vi "getGain.vi"(6 "Delay between send and receive [ms]":i32=100, 8 "error in (no error)":errorcluster, 11 "CCD in":refnum<class "CCD.lvclass">) -> (0 "error out":errorcluster, 1 "token":i32, 2 "info":string, 3 "CCD out":refnum<class "CCD.lvclass">)   [LabVIEW 2023, in "CCD.lvclass"]
doc: "Gets the current gain token and the associated description information for the gain token. Gain tokens and their descriptions are part of the CCD configuration information. See ccd_getConfig command.\nFor example:\n\n\"gains\": [\n {\n \"info\": \"Best Dynamic Range\",\n \"token\": 1\n },\n {\n \"info\": \"High Sensitivity\",\n \"token\": 2\n },\n {\n \"info\": \"High Light\",\n \"token\": 0\n }\n]"
uses:
  CCD.lvclass
  CCD.lvclass/CCD.ctl
  20f7d3bd-08ac-4524-9bed-df36c1da25a0.vi
  a21955fc-e3a0-4e36-8495-41f1bfac7860.vi
  GenericDevice/GenericDevice.lvclass
  Gain.ctl
panel:
  # "Connector Pane"
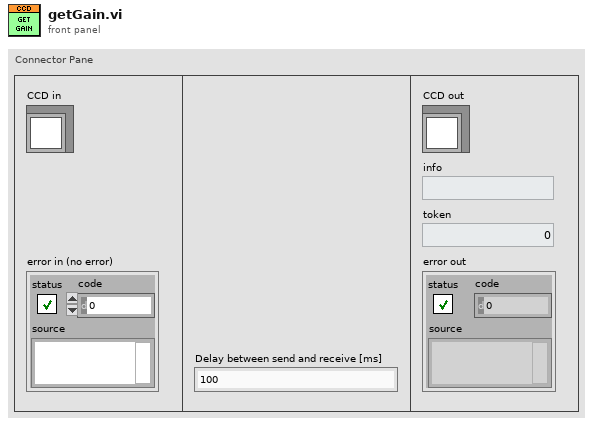
[diagram p1: front panel]
types:
  T1 = typedef "CCD.lvclass/Gain.ctl" = cluster{"info":string, "token":i32}
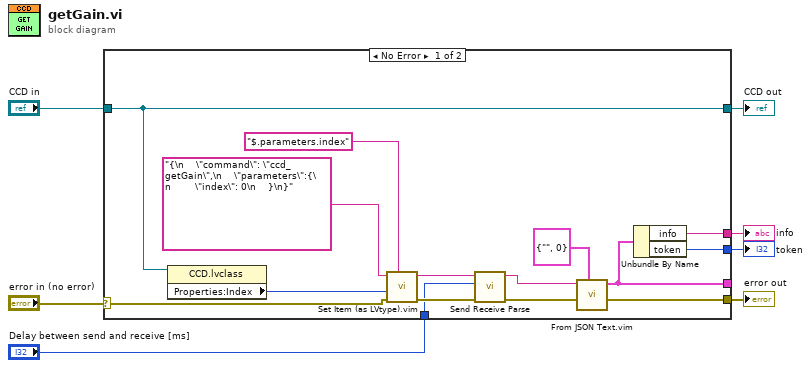
[diagram p0: block diagram]
diagram:
  n1 = case shown="No Error" "error in (no error)" {
    selector: "error in (no error)" -> [w18 w24]
    tunnel: [w17 w24] -> w6
    tunnel: [w20 w23] -> w4
    tunnel: "CCD in" -> [w20 w23]
    tunnel: [w13 _] -> _
    tunnel: [w12 _] -> w3
    tunnel: [w10 _] -> w1
    tunnel: "Delay between send and receive [ms]" -> [w11 _]
    frame No Error {
      n2 = property class="CCD.lvclass"(reference=w20) -> ("Properties:Index"=w19:i32)  [unwired: 1 in, 2 out]
      n3 = call "Set Item (as LVtype).vim"("$Path or Item Name"="$.parameters.index", "error in (no error)"=w18, "Anything"=w19, "JSON"="{\n    \"command\": \"ccd_getGain\",\n    \"parameters\":{\n        \"index\": 0\n    }\n}") -> ("error out"=w14:errorcluster, "<JSON>"=w8:string)  [unwired: 4 in, 1 out]
      n4 = call "Send Receive Parse.vi"("error in"=w14, "Delay between send and receive [ms]"=w11, "<JSON>"=w8) -> ("error out"=w15:errorcluster, "results-JSON string"=w16:string)  [unwired: 6 in, 1 out]
      n5 = call "From JSON Text.vim"("Data Type and Default Value"=T1 {"info"="", "token"=0} ("gains"), "error in (no error)"=w15, "JSON"=w16) -> ("error out"=w17:errorcluster, "Data out"=w13:T1)  [unwired: 7 in]
      n6 = Unbundle By Name(w13) -> ("info"=w12:string, "token"=w10:i32)
    }
    frame Error {
    }
  }
  "error out" <- w6
  "CCD out" <- w4
  "info" <- w3
  "token" <- w1
